vi "No heat-PID.vi"(9 "dt out (s)":dbl, 10 "setpoint":dbl, 11 "PID gains z1":T1) -> (2 "output cluster":cluster{"output":dbl} {"output" scale=0.0..100.0}, 3 "appended array":digitalwaveform[](array[waveform]))   [LabVIEW 2020]
uses:
  <vilib>/Waveform/DWDTOps.llb/DWDT Analog to Digital.vi
  <vilib>/addons/control/pid/NI_PID_autopid.lvlib
  <vilib>/measure/NI_MABase.lvlib
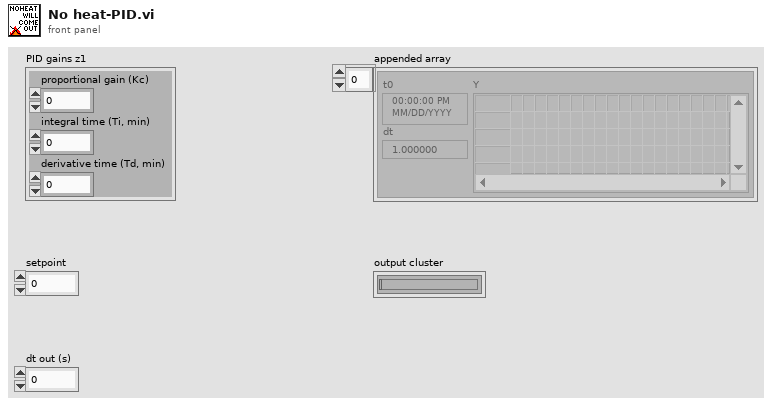
[diagram p1: front panel]
types:
  T1 = cluster{"proportional gain (Kc)":dbl, "integral time (Ti, min)":dbl, "derivative time (Td, min)":dbl}
  T2 = enum16{"Sine Wave", "Triangle Wave", "Square Wave", "Sawtooth Wave"}
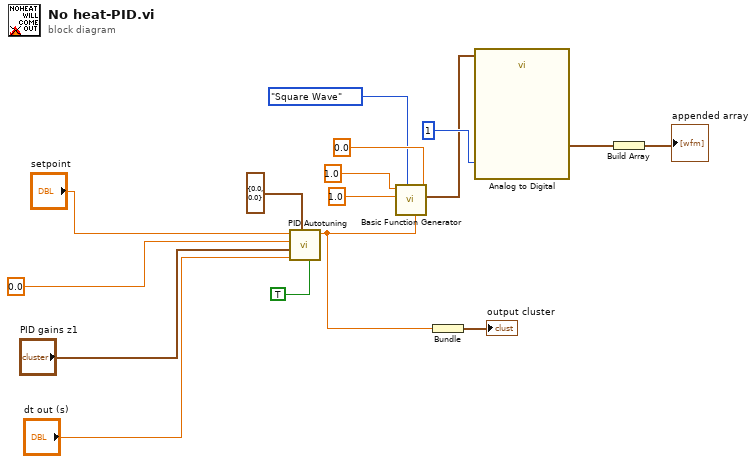
[diagram p0: block diagram]
diagram:
  n1 = call <vilib>:"PID Autotuning.vi"("autotune? (F)"=TRUE, "output range"=cluster{"output high":dbl, "output low":dbl} {"output high"=0.0, "output low"=0.0}, "dt (s)"="dt out (s)", "PID gains"="PID gains z1", "process variable"=0.0, "setpoint"="setpoint") -> ("output"=w7:dbl)  [unwired: 2 in, 3 out]
  n2 = call <vilib>:"Basic Function Generator.vi"("offset"=0.0, "square wave duty cycle (%)"=w7, "signal type"=T2."Square Wave", "amplitude"=1.0, "frequency"=1.0) -> ("signal out"=w8:waveform(dbl))  [unwired: 4 in, 2 out]
  n3 = Bundle("output"=w7) -> (→"output cluster":cluster{"output":dbl})  [unwired: 1 in]
  n4 = call-poly <vilib>:"Analog to Digital.vi"("resolution (16 bit)"=1, "analog waveform"=w8) -> ("digital waveform"=w12:digitalwaveform)  [unwired: 6 in, 3 out]
  n5 = Build Array(w12) -> (→"appended array":digitalwaveform[])
